vi "Create Translation Matrix.vi"(9 "z":sgl, 10 "y":sgl, 11 "x":sgl) -> (3 "Translation Matrix":sgl[][](array[numeric]))   [LabVIEW 2020, in "3D.lvlib"]
uses:
  3D.lvlib
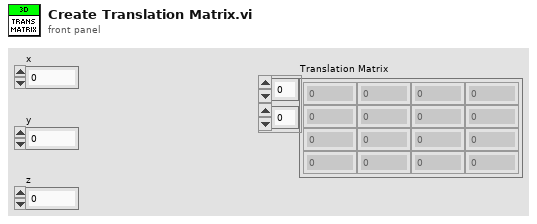
[diagram p1: front panel]
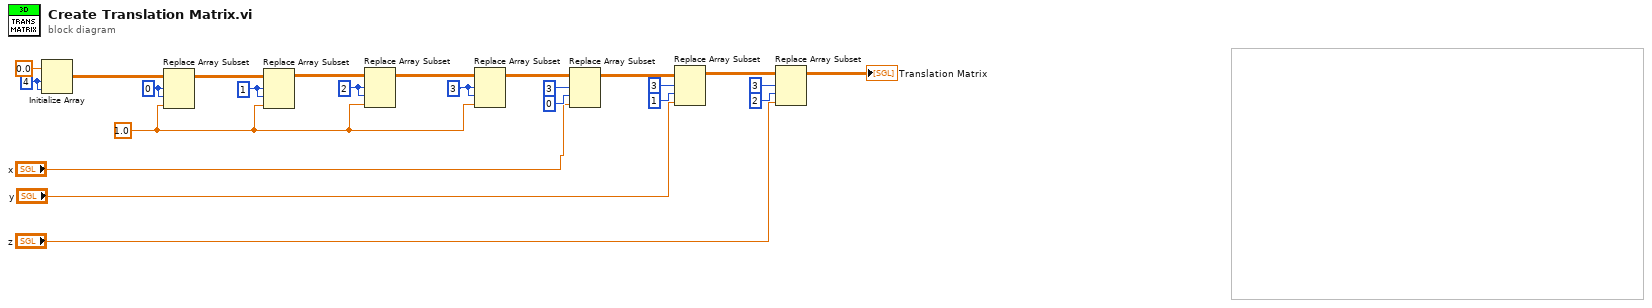
[diagram p0: block diagram]
diagram:
  w10 = sgl 1.0 ("new element/subarray")
  w11 = 3 ("index (row)")
  w12 = 2 ("index (row)")
  w13 = 1 ("index (row)")
  w22 = 0 ("index (row)")
  w23 = 4 ("dimension size")
  n1 = Initialize Array(sgl 0.0 ("element"), w23, w23) -> (w14:sgl[][])
  n2 = Replace Array Subset(array=w14, new element=w10, index (row)=w22, index (col)=w22) -> (w21:sgl[][])
  n3 = Replace Array Subset(array=w21, new element=w10, index (row)=w13, index (col)=w13) -> (w20:sgl[][])
  n4 = Replace Array Subset(array=w20, new element=w10, index (row)=w12, index (col)=w12) -> (w19:sgl[][])
  n5 = Replace Array Subset(array=w19, new element=w10, index (row)=w11, index (col)=w11) -> (w18:sgl[][])
  n6 = Replace Array Subset(array=w18, new element="x", index (row)=3, index (col)=0 ("index (row)")) -> (w16:sgl[][])
  n7 = Replace Array Subset(array=w16, new element="y", index (row)=3, index (col)=1 ("index (row)")) -> (w5:sgl[][])
  n8 = Replace Array Subset(array=w5, new element="z", index (row)=3, index (col)=2 ("index (row)")) -> (→"Translation Matrix":sgl[][])
